vi "Trajectory_Controller.vi"(0 "Error In":errorcluster, 1 "reset":dbl, 3 "Abort Trajectory":bool, 5 "Configuration":T1={"Accelerometer Bias"={"X (m/s)"=0.0, "Y (m/s)"=0.0, "Z (m/s)"=0.0}, "Gyroscope Bias"={"X (m/s)"=0.0, "Y (m/s)"=0.0, "Z (m/s)"=0.0}, "Steering Motor Gear Ratio"=611.0, "Steering Pully Gear Ratio"=1.0, "Steering Encoder CPR"=500.0, "Steering Motor Max RPM"=4000.0, "Wheelbase (m)"=1.12, "Fork Angle (rad)"=1.3, "Balancing Controller"={"Kp (/s)"=1.0, "Kd (1)"=1.0}, "Max Allowed Steering Angle (rad)"=0.7, "Task Periods"={"Emergency Stop (us)"=10000, "IMU (us)"=10000, "Steering Motor Encoder (us)"=10000, "State Estimator (us)"=10000, "Balancing Controller (us)"=10000, "GNSS (us)"=10000, "Logging (us)"=50000, "Drive Motor (us)"=100000, "Visualization (us)"=50000, "Reaction Wheel (us)"=10000}, "Drive Motor Gear Ratio"=0.7, "lr"=0.0, "lf"=0.0, "lambda"=0.0, "k1"=0.0, "k2"=0.0, "e1_max"=0.0, "Ad_t"=0.0, "Bd_t"=0.0, "C_t"=0.0, "D_t"=0.0, "Wheel radius"=0.311}, 7 "State Estimate In":refnum<data-value>, 9 "Reset and Init trajectory":bool, 11 "RefTraj in":refnum<data-value>, 12 "Trajectory In":refnum<data-value>, 13 "Measurement In":refnum<data-value>) -> (2 "Measurement Out":refnum<data-value>, 6 "Error out":errorcluster, 10 "Trajectory Out":refnum<data-value>, 14 "E1 limit":bool, 15 "E2 limit":bool)   [LabVIEW 2021]
uses:
  State Estimator/State Estimate.ctl
  Trajectory_Control.ctl
  Configuration/Configuration.ctl
  State Estimator/Measurements.ctl
  IMU/IMU Data.ctl
  Steering Motor Encoder/Steering Motor Encoder Data.ctl
  GNSS/GNSS Data.ctl
panel:
  out "lat_con":dbl
  out "head con":dbl
  out "delta":dbl
  out "State Estimate In 2":refnum<data-value>
  out "RefTraj out":refnum<data-value>
  out "size(s)":i32[](array[numeric])
  out "error2":dbl
  out "error1":dbl
  out "Rollref":dbl
  out "Closestpoint":dbl
  in  "path in":path=path "libtrajectory_controller.so"
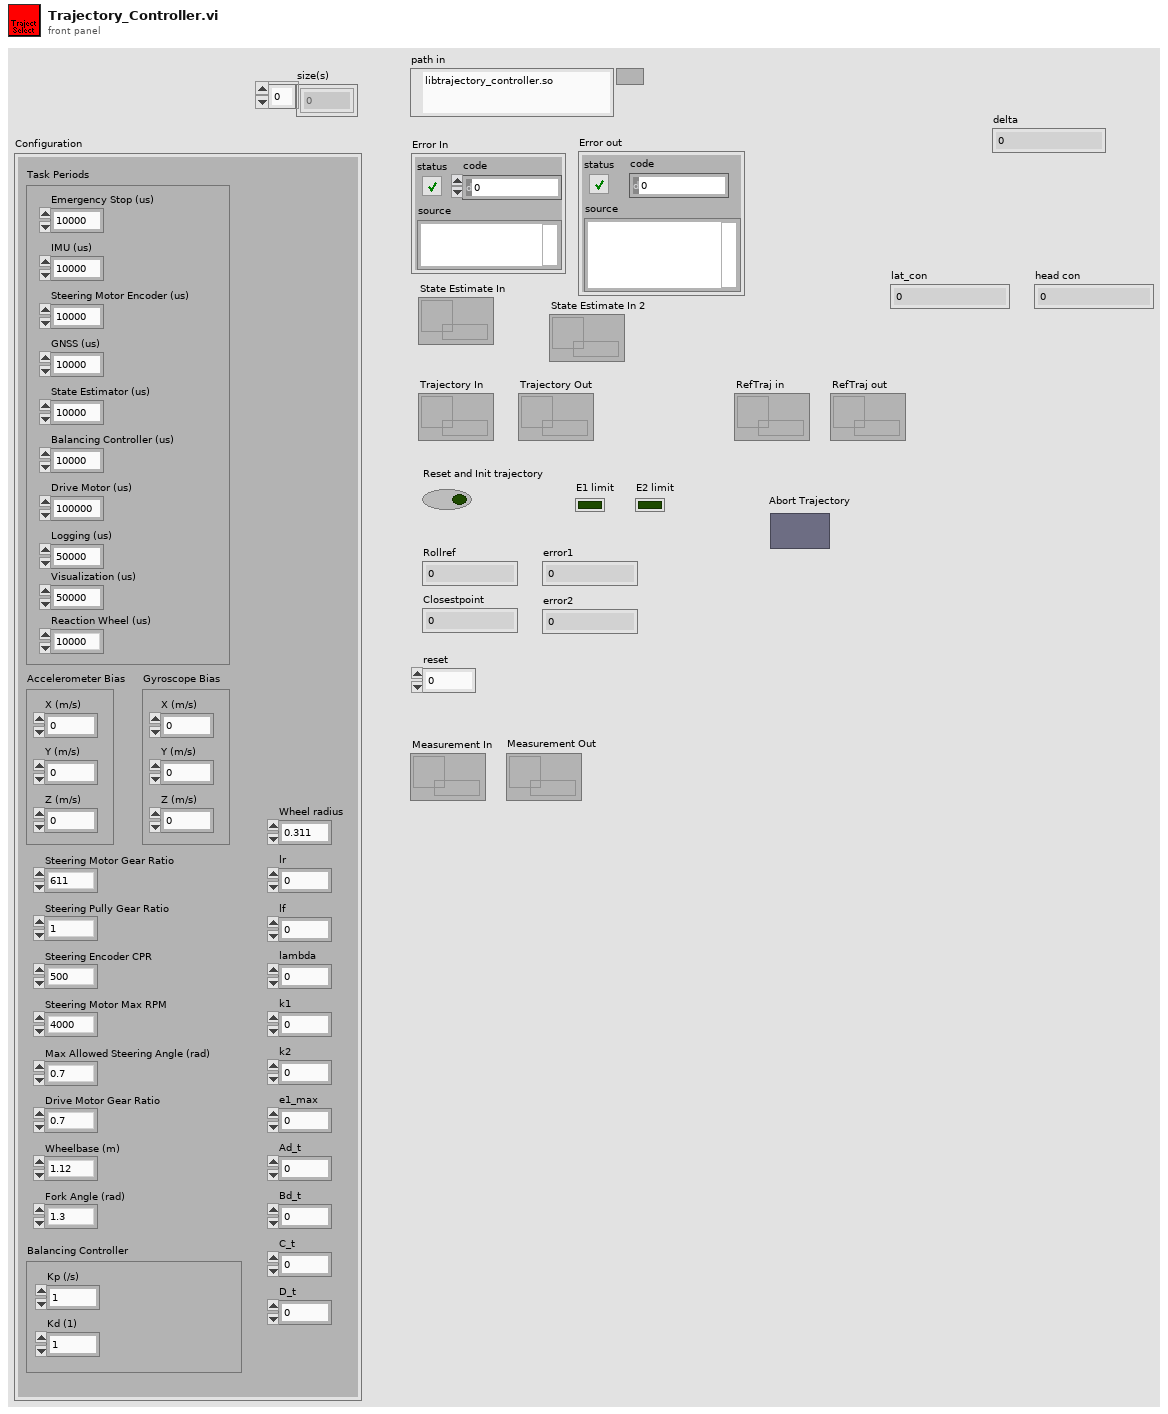
[diagram p1: front panel]
types:
  T1 = typedef "Configuration.ctl" = cluster{"Accelerometer Bias":cluster{"X (m/s)":dbl, "Y (m/s)":dbl, "Z (m/s)":dbl}, "Gyroscope Bias":cluster{"X (m/s)":dbl, "Y (m/s)":dbl, "Z (m/s)":dbl}, "Steering Motor Gear Ratio":dbl, "Steering Pully Gear Ratio":dbl, "Steering Encoder CPR":dbl, "Steering Motor Max RPM":dbl, "Wheelbase (m)":dbl, "Fork Angle (rad)":dbl, "Balancing Controller":cluster{"Kp (/s)":dbl, "Kd (1)":dbl}, "Max Allowed Steering Angle (rad)":dbl, "Task Periods":cluster{"Emergency Stop (us)":i64, "IMU (us)":i64, "Steering Motor Encoder (us)":i64, "State Estimator (us)":i64, "Balancing Controller (us)":i64, "GNSS (us)":i64, "Logging (us)":i64, "Drive Motor (us)":i64, "Visualization (us)":i64, "Reaction Wheel (us)":i64}, "Drive Motor Gear Ratio":dbl, "lr":dbl, "lf":dbl, "lambda":dbl, "k1":dbl, "k2":dbl, "e1_max":dbl, "Ad_t":dbl, "Bd_t":dbl, "C_t":dbl, "D_t":dbl, "Wheel radius":dbl}
  T2 = typedef "Trajectory_Control.ctl" = cluster{"Rollref":dbl, "Closestpoint":dbl, "Error1":dbl, "Error2":dbl, "Dpsiref_cont":dbl, "Lateral_cont":dbl, "Heading_cont":dbl, "Reset_traj":dbl, "Iteration":dbl, "E1 limit":u32, "E2 limit":u32}
  T3 = typedef "Measurements.ctl" = cluster{"IMU Data":T4, "Steering Motor Encoder Data":T5, "GNSS Data":T6}
  T4 = typedef "IMU Data.ctl" = cluster{"Gyroscope":cluster{"X (rad/s)":dbl, "Y (rad/s)":dbl, "Z (rad/s)":dbl}, "Accelerometer":cluster{"X (m/s^2)":dbl, "Y (m/s^2)":dbl, "Z (m/s^2)":dbl}, "Flag IMU":dbl}
  T5 = typedef "Steering Motor Encoder Data.ctl" = cluster{"Encoder Position (counts)":i32, "Steering Angle (rad)":dbl, "Flag Steering Encoder":dbl}
  T6 = typedef "GNSS Data.ctl" = cluster{"Latitude (rad)":dbl, "Longitude (rad)":dbl, "Altitude (m)":dbl, "Speed (m/s)":dbl, "Heading (rad)":dbl, "Fix Quality":i32, "Number of Satellites":i32, "Latitude (deg)":dbl, "Longitude (deg)":dbl, "Flag GNSS":dbl}
  T7 = typedef "State Estimate.ctl" = cluster{"X (m)":dbl, "Y (m)":dbl, "Psi (rad)":dbl, "Roll (rad)":dbl, "Roll Rate (rad/s)":dbl, "delta":dbl, "velocity":dbl, "Iterations":dbl}
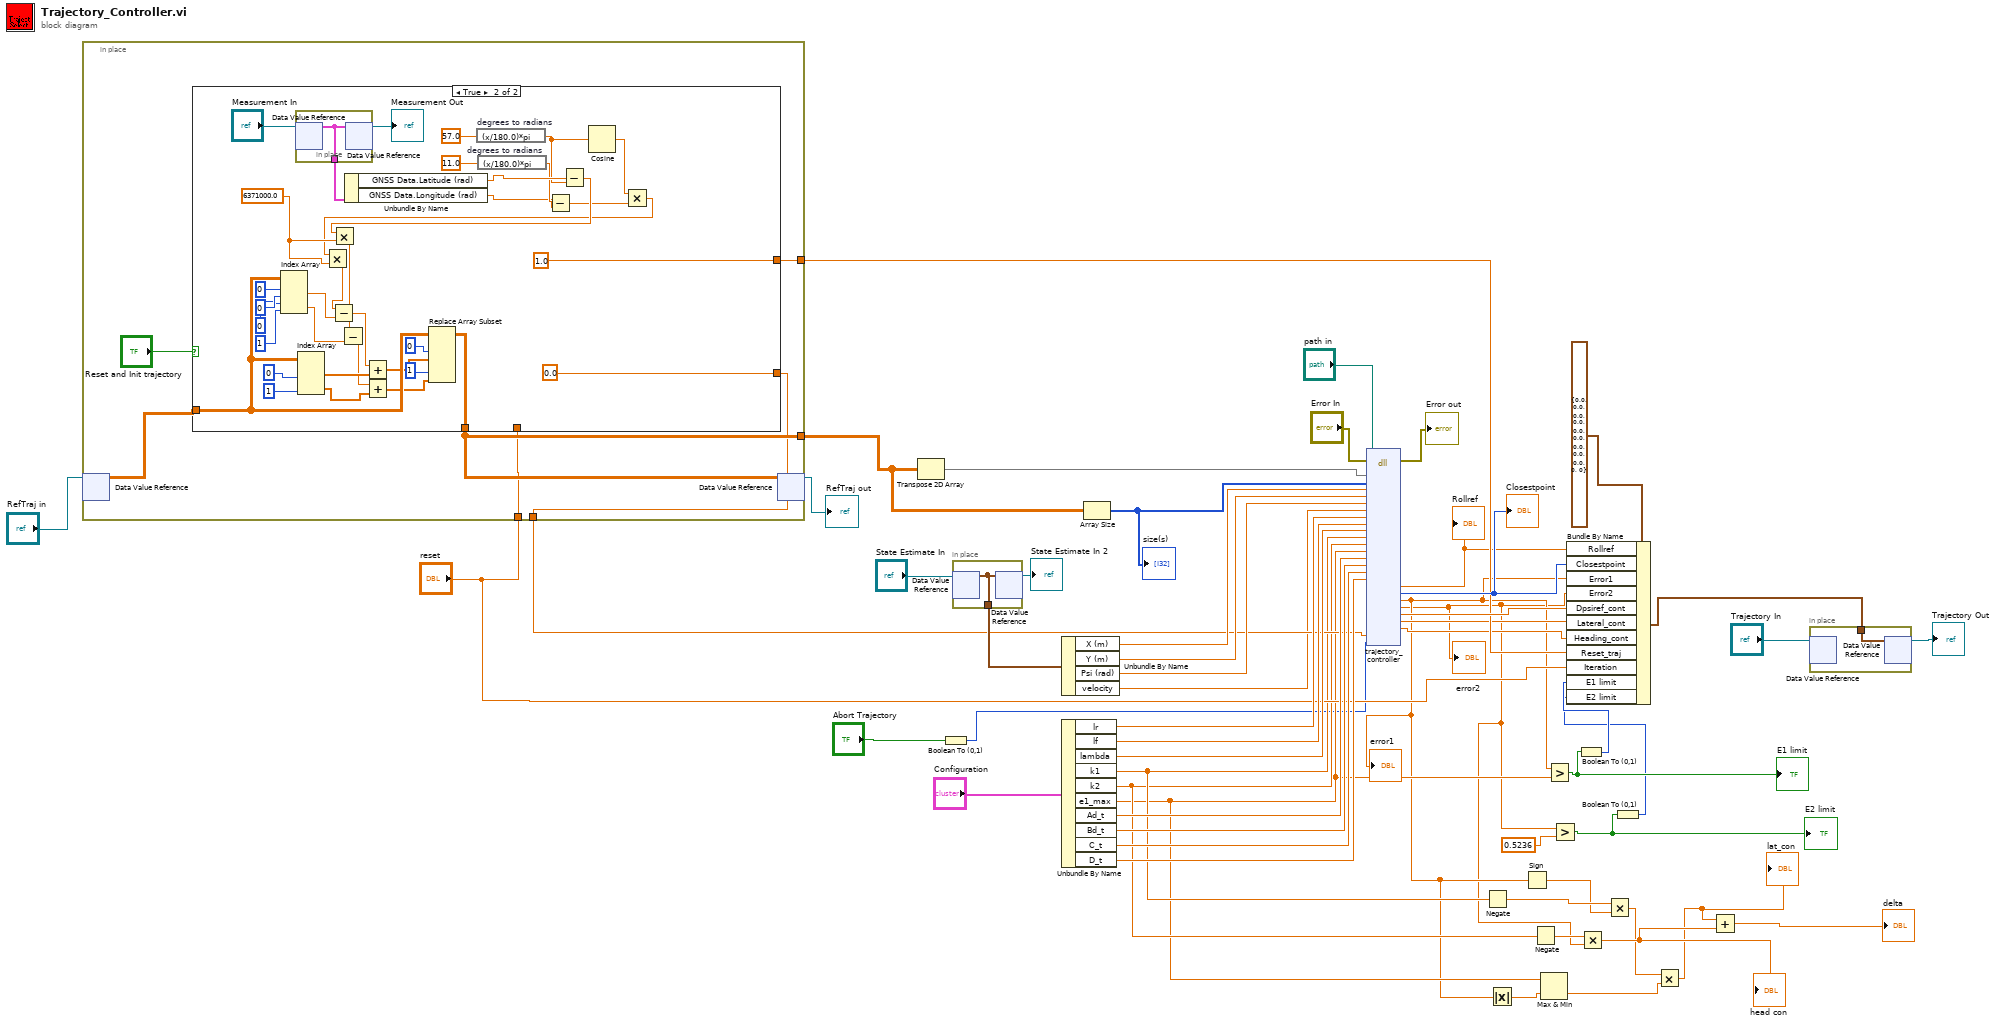
[diagram p0: block diagram]
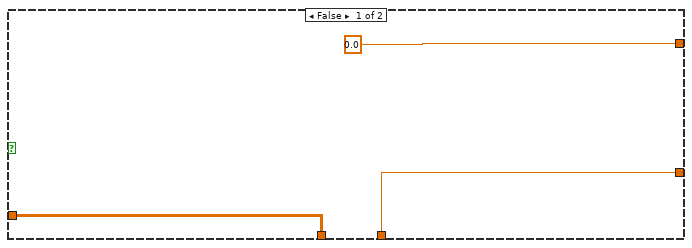
[diagram p2: hidden frame]
diagram:
  n1 = in-place {
    in-place-border: [w60] -> w29
    in-place-border: [w62] -> w32
    in-place-border: [w58] -> w31
    in-place-border: "reset" -> [w57]
    n2 = in-place-dvr #1("RefTraj in") -> (w61:dbl[][])  [unwired: 1 out]
    n3 = case shown="True" "Reset and Init trajectory" {
      tunnel: [w63 0.0] -> w60
      tunnel: [w65 w83] -> w62
      tunnel: w61 -> [w65 w93]
      tunnel: [0.0 1.0] -> w58
      tunnel: w57 -> [w63 _]
      frame False {
      }
      frame True {
        w95 = 6371000.0
        n4 = Index Array(array=w93, index (row) #1=0, index (col) #1=0, index (row) #2=0, index (col) #2=1) -> (element #1=w67:dbl, element #2=w88:dbl)
        n5 = in-place {
          in-place-border: [w102] -> w98
          n6 = in-place-dvr #2("Measurement In") -> (w102:T3)  [unwired: 1 out]
          n7 = in-place-dvr #2(w102) -> (→"Measurement Out":refnum<data-value>)  [unwired: 1 out]
        }
        n8 = Index Array(array=w93, index (col) #1=0, index (col) #2=1) -> (element #1=w96:dbl[], element #2=w85:dbl[])  [unwired: 2 in]
        n9 = Unbundle By Name(w98) -> ("GNSS Data.Latitude (rad)"=w77:dbl, "GNSS Data.Longitude (rad)"=w74:dbl)
        n10 = expression code="(x/180.0)*pi" "degrees to radians"(57.0 ("y")) -> (w72:dbl)
        n11 = expression code="(x/180.0)*pi" "degrees to radians"(11.0 ("y")) -> (w75:dbl)
        n12 = Subtract(x=w74, y=w75) -> (x-y=w70:dbl)
        n13 = Subtract(x=w77, y=w72) -> (x-y=w73:dbl)
        n14 = Multiply(x=w73, y=w95) -> (x*y=w94:dbl)
        n15 = Subtract(x=w94, y=w88) -> (x-y=w86:dbl)
        n16 = Add(x=w86, y=w85) -> (x+y=w84:dbl[])
        n17 = Cosine(x=w72) -> (cos(x)=w71:dbl)
        n18 = Multiply(x=w71, y=w70) -> (x*y=w69:dbl)
        n19 = Multiply(x=w69, y=w95) -> (x*y=w68:dbl)
        n20 = Subtract(x=w68, y=w67) -> (x-y=w97:dbl)
        n21 = Add(x=w97, y=w96) -> (x+y=w87:dbl[])
        n22 = Replace Array Subset(array=w93, new element #1=w87, index (col) #1=0, new element #2=w84, index (col) #2=1) -> (w83:dbl[][])  [unwired: 2 in]
      }
    }
    n23 = in-place-dvr #1(w62) -> (→"RefTraj out":refnum<data-value>)  [unwired: 1 out]
  }
  n24 = Transpose 2D Array(2D array=w32) -> (transposed array=w33:dbl[][])
  n25 = Boolean To (0,1)(Boolean="Abort Trajectory") -> (0, 1=w1:i16)
  n26 = in-place {
    in-place-border: [w103] -> w54
    n27 = in-place-dvr #3("State Estimate In") -> (w103:T7)  [unwired: 1 out]
    n28 = in-place-dvr #3(w103) -> (→"State Estimate In 2":refnum<data-value>)  [unwired: 1 out]
  }
  n29 = Unbundle By Name(w54) -> ("X (m)"=w53:dbl, "Y (m)"=w52:dbl, "Psi (rad)"=w51:dbl, "velocity"=w25:dbl)
  n30 = Unbundle By Name("Configuration") -> ("lr"=w45:dbl, "lf"=w44:dbl, "lambda"=w43:dbl, "k1"=w24:dbl, "k2"=w23:dbl, "e1_max"=w17:dbl, "Ad_t"=w42:dbl, "Bd_t"=w41:dbl, "C_t"=w40:dbl, "D_t"=w39:dbl)
  n31 = Array Size(array=w32) -> (size(s)=w34:i32[])
  "size(s)" <- w34
  n32 = dll-call lib="libtrajectory_controller.so" fn="trajectory_controller"(path in="path in", error in="Error In", "Traj"=w33, "traj_size"=w34, "X"=w53, "Y"=w52, "Psi"=w51, "v"=w25, "lr"=w45, "lf"=w44, "lambda"=w43, "k1"=w24, "k2"=w23, "e1max"=w17, "Adt"=w42, "Bdt"=w41, "Ct"=w40, "Dt"=w39, "Reset"=w29, "abort"=w1) -> (error out=→"Error out":errorcluster, "Rollref"=w28:dbl, "Closestpoint"=w38:i32, "error1"=w10:dbl, "error2"=w9:dbl, "dpsiref_cont"=w37:dbl, "Lateral_cont"=w11:dbl, "Heading_cont"=w12:dbl)  [unwired: 27 in, 1 out]
  "Closestpoint" <- w38
  "Rollref" <- w28
  "error1" <- w10
  "error2" <- w9
  n33 = Negate(x=w24) -> (-x=w22:dbl)
  n34 = Absolute Value(x=w10) -> (abs(x)=w16:dbl)
  n35 = Sign(1:w10) -> (0:w18:dbl)
  n36 = Negate(x=w23) -> (-x=w21:dbl)
  n37 = Max & Min(x=w17, y=w16) -> (min(x,y)=w15:dbl)  [unwired: 1 out]
  n38 = Greater?(x=w10, y=w17) -> (0:w5:bool)
  "E1 limit" <- w5
  n39 = Greater?(x=w9, y=0.5236) -> (0:w6:bool)
  "E2 limit" <- w6
  n40 = Boolean To (0,1)(Boolean=w5) -> (0, 1=w4:i16)
  n41 = Multiply(x=w21, y=w9) -> (x*y=w20:dbl)
  "head con" <- w20
  n42 = Multiply(x=w22, y=w18) -> (x*y=w14:dbl)
  n43 = Boolean To (0,1)(Boolean=w6) -> (0, 1=w3:i16)
  n44 = Bundle By Name(cluster=T2 {"Rollref"=0.0, "Closestpoint"=0.0, "Error1"=0.0, "Error2"=0.0, "Dpsiref_cont"=0.0, "Lateral_cont"=0.0, "Heading_cont"=0.0, "Reset_traj"=0.0, "Iteration"=0.0, "E1 limit"=0, "E2 limit"=0} ("Trajectory (Debug)"), "Rollref"=w28, "Closestpoint"=w38, "Error1"=w10, "Error2"=w9, "Dpsiref_cont"=w37, "Lateral_cont"=w11, "Heading_cont"=w12, "Reset_traj"=w31, "Iteration"="reset", "E1 limit"=w4, "E2 limit"=w3) -> (w7:T2)
  n45 = Multiply(x=w14, y=w15) -> (x*y=w13:dbl)
  "lat_con" <- w13
  n46 = Add(x=w13, y=w20) -> (x+y=→"delta":dbl)
  n47 = in-place {
    in-place-border: w7 -> [w104]
    n48 = in-place-dvr #4("Trajectory In") -> ()  [unwired: 2 out]
    n49 = in-place-dvr #4(w104) -> (→"Trajectory Out":refnum<data-value>)  [unwired: 1 out]
  }
